vi "Get Greeting Ref.vi"(8 "error in (no error)":errorcluster, 11 "WebSocket Test UI Refs in":refnum<class "WebSocket Test UI Refs.lvclass">) -> (0 "error out":errorcluster, 2 "Last Greeting":refnum<vi>, 3 "WebSocket Test UI Refs out":refnum<class "WebSocket Test UI Refs.lvclass">)   [LabVIEW 2020, in "WebSocket Test UI Refs.lvclass"]
uses:
  WebSocket Test UI Refs.lvclass
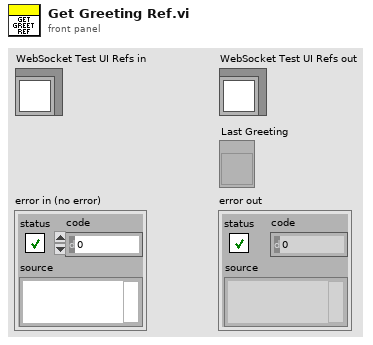
[diagram p1: front panel]
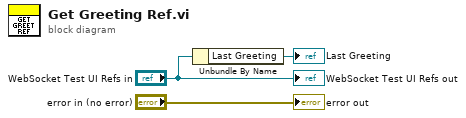
[diagram p0: block diagram]
diagram:
  n1 = Unbundle By Name("WebSocket Test UI Refs in") -> ("Last Greeting"=→"Last Greeting":refnum<vi>)
  "error out" <- "error in (no error)"
  "WebSocket Test UI Refs out" <- "WebSocket Test UI Refs in"
